vi "ConfigChannel.vi"(8 "error in":T6, 11 "Channel Cluster":T1={"Channel"=1, "Source"=-2147483648, "Average"=-2147483648, "SampleTime [us]"=-inf, "Trigger"=-2147483648} {"Trigger" items=["[read only]"=-2147483648, "Disabled"=0, "Scanner"=1, "Permanent"=2, "Spectroscopy 1"=3, "Spectroscopy 2"=4, "Spectroscopy 3"=5, "Calibration"=6, "Trigger"=7, "Every"=8, "Command"=9, "2nd Pass"=13, "Step Scan"=16]; "Average" items=["[read only]"=-2147483648, "no"=0, "yes"=1]; "Source" items=["[read only]"=-2147483648, "ADC 1"=0, "ADC 2"=1, "ADC 3"=2, "ADC 4"=3, "ADC 5"=4, "ADC 6"=5, "HF 1 Out"=7, "HF 1 df"=8, "z out"=9, "HF 1"=12, "HF 1 Ampl."=13, "HF 1 Phase"=14, "LF LockIn Ampl"=16, "LF LockIn Phase"=17, "z out inv"=18, "counter"=23, "Crosslink 1"=29, "Crosslink 2"=30, "Pos X"=31, "Pos Y"=32]; "Channel" items=["Channel 0", "Channel 1", "Channel 2", "Channel 3", "Channel 4", "Channel 5", "Channel 6", "Channel 7", "Channel 8", "Channel 9", "Channel 10", "Channel 11", "Channel 12", "Channel 13"]}) -> (0 "error out":T6, 3 "Output Cluster":T1={"Channel"=1, "Source"=1, "Average"=0, "SampleTime [us]"=-inf, "Trigger"=0} {"Trigger" items=["[read only]"=-2147483648, "Disabled"=0, "Scanner"=1, "Permanent"=2, "Spectroscopy 1"=3, "Spectroscopy 2"=4, "Spectroscopy 3"=5, "Calibration"=6, "Trigger"=7, "Every"=8, "Command"=9, "2nd Pass"=13, "Step Scan"=16]; "Average" items=["[read only]"=-2147483648, "no"=0, "yes"=1]; "Source" items=["[read only]"=-2147483648, "ADC 1"=0, "ADC 2"=1, "ADC 3"=2, "ADC 4"=3, "ADC 5"=4, "ADC 6"=5, "HF 1 Out"=7, "HF 1 df"=8, "z out"=9, "HF 1"=12, "HF 1 Ampl."=13, "HF 1 Phase"=14, "LF LockIn Ampl"=16, "LF LockIn Phase"=17, "z out inv"=18, "counter"=23, "Crosslink 1"=29, "Crosslink 2"=30, "Pos X"=31, "Pos Y"=32]; "Channel" items=["Channel 0", "Channel 1", "Channel 2", "Channel 3", "Channel 4", "Channel 5", "Channel 6", "Channel 7", "Channel 8", "Channel 9", "Channel 10", "Channel 11", "Channel 12", "Channel 13"]})   [LabVIEW 2016]
doc: "Prepares a channel for data reception. The channel cluster contains:\n- channel (integer)[0 to 13]\n- trigger (integer) [0 -- disabled; 1 -- scanner; 2 -- permanent; 3,4,5,6 -- spectroscopy 0,1,2,3; 9 -- command]\n- source (integer)[0-5 -- ADC 0-5; 7 -- aexc; 8 -- fexc; 9 -- zOut; 12 -- signal; 13 -- ampl; 14 -- phase; 15 -- mampl; 17 -- mphase; 18 - zoutinv; 20 -- ADCext_min; 21 -- ADCext_max]\n- average (integer)[0 to 1]\n- sample time (float)\nThe 'channel' is used to identify the data channel later. 'Trigger' specifies the expected data format coming from the 'source'. If the trigger was set to permanent, a 'sample time' may be stated over which is averaged if the 'average' flag has been set.\nIf you want to get the current settings of a specific channel, please use getChannelConfig.vi."
uses:
  Controls/Channel_Parameters.ctl
  Controls/Channel_Selection.ctl
  Controls/Channel-Source_Selection.ctl
  Controls/Average_Selection.ctl
  Controls/Trigger_Selection.ctl
  Controls/Error_Out.ctl
  Files_ASC500/DLL/ASC500_RemoteControlV27.dll
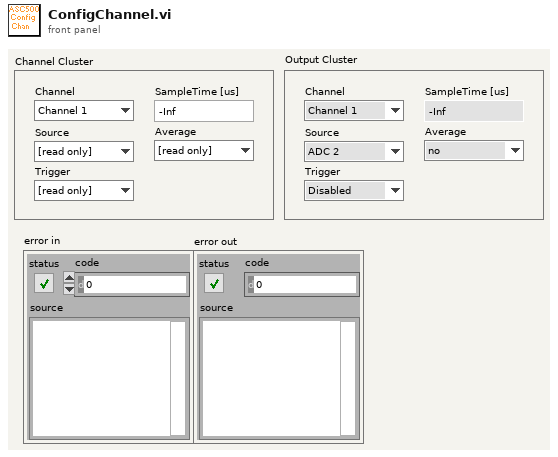
[diagram p1: front panel]
types:
  T1 = typedef "Channel_Parameters.ctl" = cluster{"Channel":T2, "Source":T3, "Average":T4, "SampleTime [us]":sgl, "Trigger":T5}
  T2 = typedef "Channel_Selection.ctl" = i32
  T3 = typedef "Channel-Source_Selection.ctl" = i32
  T4 = typedef "Average_Selection.ctl" = i32
  T5 = typedef "Trigger_Selection.ctl" = i32
  T6 = typedef "Error_Out.ctl" = errorcluster
  T7 = cluster{"Channel":i32, "Trigger":i32, "Source":i32, "Average":i32, "SampleTime":sgl}
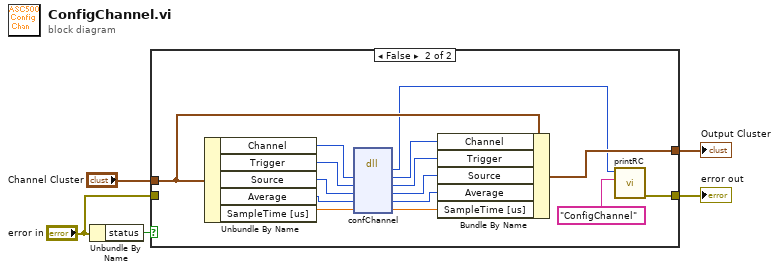
[diagram p0: block diagram]
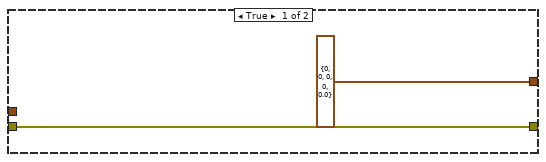
[diagram p2: hidden frame]
diagram:
  n1 = Unbundle By Name("error in") -> ("status"=w5:bool)
  n2 = case shown="False" w5 {
    tunnel: [w6 w10] -> w4
    tunnel: "Channel Cluster" -> [_ w17]
    tunnel: [T7 {"Channel"=0, "Trigger"=0, "Source"=0, "Average"=0, "SampleTime"=0.0} w11] -> w2
    tunnel: "error in" -> [w6 _]
    frame True {
    }
    frame False {
      n3 = Unbundle By Name(w17) -> ("Channel"=w22:T2, "Trigger"=w21:T5, "Source"=w20:T3, "Average"=w19:T4, "SampleTime [us]"=w18:sgl)
      n4 = dll-call lib="G:/SCMOperations/Share/ELE/Produkt Information/ASC500/04 Remote Control/02 development versions/2018Nov06/Files_ASC500/DLL/ASC500_RemoteControlV27.dll" fn="confChannel"("Channel"=w22, "Trigger"=w21, "Source"=w20, "Average"=w19, "SampleTime"=w18) -> ("return type"=w9:i32, "Channel"=w16:i32, "Trigger"=w15:i32, "Source"=w14:i32, "Average"=w13:i32, "SampleTime"=w12:sgl)  [unwired: 3 in, 2 out]
      n5 = Bundle By Name(cluster=w17, "Channel"=w16, "Trigger"=w15, "Source"=w14, "Average"=w13, "SampleTime [us]"=w12) -> (w11:T1)
      n6 = call "printRC.vi"("additional information"="ConfigChannel", "RC"=w9) -> ("error out"=w10:T6)  [unwired: 9 in]
    }
  }
  "error out" <- w4
  "Output Cluster" <- w2
